vi "NextObject.vi"(8 "error in (no error)":errorcluster, 11 "reference in":refnum<class "ArrayIterator.lvclass">) -> (0 "error out":errorcluster, 2 "BrowerComponent":refnum<class "BrowerComponent.lvclass">, 3 "reference out":refnum<class "ArrayIterator.lvclass">)   [LabVIEW 2015, in "ArrayIterator.lvclass"]
uses:
  ArrayIterator.lvclass
  BrowerComponent/BrowerComponent/BrowerComponent.lvclass
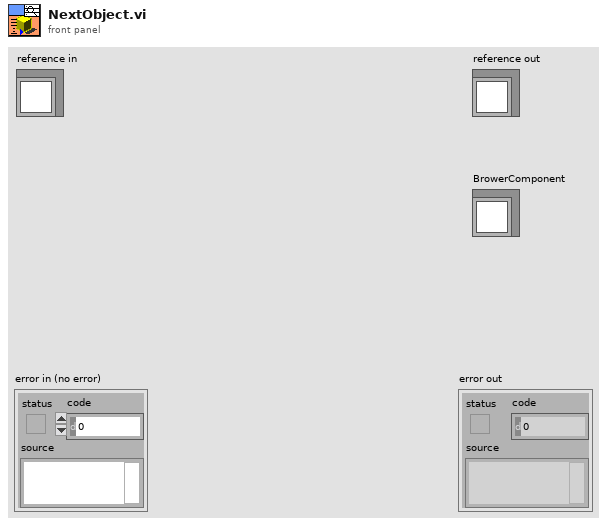
[diagram p1: front panel]
types:
  T1 = typedef "ArrayIterator.lvclass/ObjectAttributes.ctl" = cluster{"BrowerComponents":refnum<class "BrowerComponent.lvclass">[], "IndexOfComponents":i32}
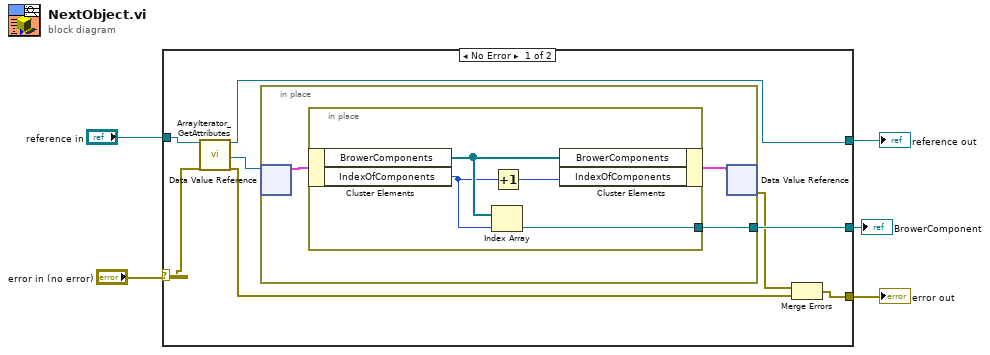
[diagram p0: block diagram]
diagram:
  n1 = case shown="No Error" "error in (no error)" {
    selector: "error in (no error)" -> [w11 w22]
    tunnel: [w6 w22] -> w4
    tunnel: "reference in" -> [w12 w21]
    tunnel: [w13 _] -> w2
    tunnel: [w9 w21] -> w1
    frame No Error {
      n2 = call "ArrayIterator_GetAttributes.vi"("reference in"=w12, "error in (no error)"=w11) -> ("reference out"=w9:refnum<class "ArrayIterator.lvclass">, "DataRef"=w10:refnum<data-value>, "error out"=w7:errorcluster)  [unwired: 14 in, 1 out]
      n3 = in-place {
        in-place-border: [w16] -> w13
        n4 = in-place-dvr #1(w10) -> (w15:T1)  [unwired: 1 out]
        n5 = in-place {
          in-place-border: [w20] -> w16
          n6 = in-place-cluster #2(w15) -> ("BrowerComponents"=w19:refnum<class "BrowerComponent.lvclass">[], "IndexOfComponents"=w18:i32)
          n7 = Index Array(array=w19, index=w18) -> (element=w20:refnum<class "BrowerComponent.lvclass">)
          n8 = Increment(x=w18) -> (x+1=w17:i32)
          n9 = in-place-cluster #2("BrowerComponents"=w19, "IndexOfComponents"=w17) -> (w14:T1)
        }
        n10 = in-place-dvr #1(w14) -> (w8:errorcluster)  [unwired: 1 out]
      }
      n11 = Merge Errors(w8, w7) -> (w6:errorcluster)
    }
    frame Error {
    }
  }
  "error out" <- w4
  "BrowerComponent" <- w2
  "reference out" <- w1
